vi "ADB-LMS_Esp32.vi"(5 "Monitor Refnum":refnum<vi>, 9 "Serial PID":string, 11 "COM BLE Esp32":refnum<visa-resource-name>) -> (1 "Check  BLE":bool, 2 "CMD Monitor":string="\r\n", 3 "BLE PID Str":string, 4 "Err Open Cnt":u16)   [LabVIEW 2018]
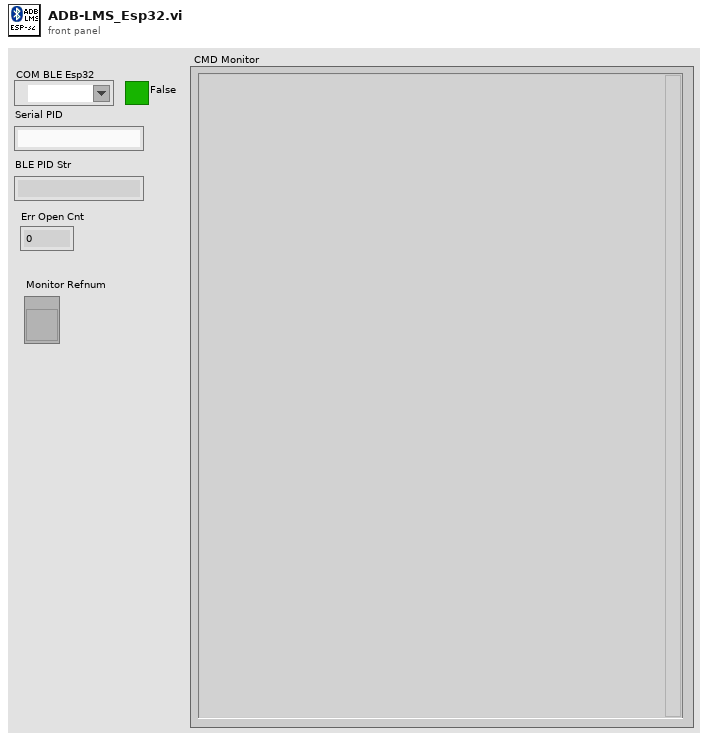
[diagram p1: front panel]
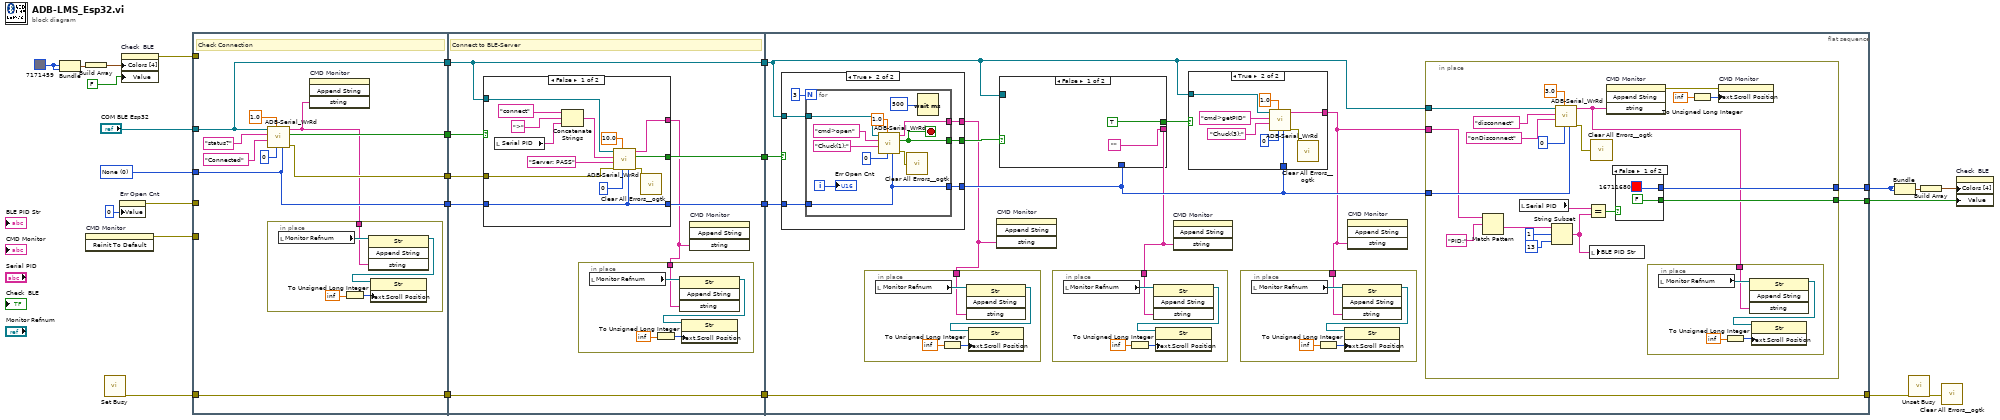
[diagram p0: block diagram]
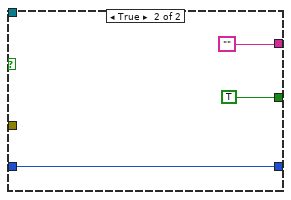
[diagram p2: hidden frame]
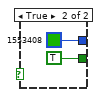
[diagram p3: hidden frame]
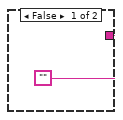
[diagram p4: hidden frame]
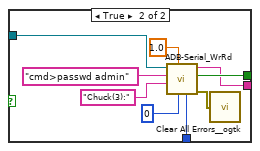
[diagram p5: hidden frame]
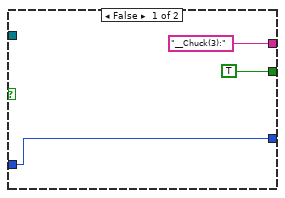
[diagram p6: hidden frame]
diagram:
  w22 = u32 7171459
  w25 = u16 0 items=["None", "XON/XOFF", "RTS/CTS", "XON/XOFF & RTS/CTS", "DTR/DSR", "XON/XOFF & DTR/DSR"] ("flow control (0:none)")
  n1 = Bundle(w22, w22) -> (w23:cluster{u32, u32})  [unwired: 1 in]
  n2 = Build Array(w23) -> (w11:cluster{u32, u32}[])
  n3 = invoke on="CMD Monitor" class="Str" method="Reinit To Default"() -> (error out=w24:errorcluster)  [unwired: 3 in, 2 out]
  n4 = call <vilib>:"Set Busy.vi"() -> ("error out"=w21:errorcluster)  [unwired: 10 in, 1 out]
  n5 = property on="Err Open Cnt" class="DigNum (strict)"("Value"=u16 0 ("Err Open Cnt")) -> (error out=w4:errorcluster)  [unwired: 2 in, 1 out]
  n6 = property on="Check  BLE" class="Bool (strict)"("Colors [4]"=w11, "Value"=FALSE ("Check  BLE")) -> (error out=w12:errorcluster)  [unwired: 2 in, 1 out]
  n7 = flat-sequence {
    tunnel: "COM BLE Esp32" -> [w31]
    tunnel: w25 -> [w29]
    tunnel: w24 -> [_]
    tunnel: w21 -> [w28]
    tunnel: [w32] -> w20
    tunnel: [w31] -> w19
    tunnel: [w30] -> w18
    tunnel: [w29] -> w17
    tunnel: [w28] -> w16
    tunnel: w12 -> [_]
    tunnel: w4 -> [_]
    tunnel: w20 -> [w49]
    tunnel: w19 -> [w44]
    tunnel: w18 -> [w48]
    tunnel: w17 -> [w47]
    tunnel: w16 -> [w45]
    tunnel: [w46] -> w15
    tunnel: [w45] -> w14
    tunnel: [w43] -> w13
    tunnel: [w44] -> w9
    tunnel: [w82] -> w3
    tunnel: w15 -> [w81]
    tunnel: w14 -> [w82]
    tunnel: w13 -> [w80]
    tunnel: w9 -> [w77]
    tunnel: [w76] -> w2
    tunnel: [w75] -> w1
    frame #0 {
      # "Check Connection"
      n8 = call "ADB-Serial_WrRd.vi"("flow control (0:none)"=w29, "Tx Deay"=u16 0, "Timeout(Sec)"=1.0, "PassString"="Connected", "Command"="status?", "ComPort"=w31) -> ("error out"=w30:errorcluster, "PASS"=w32:bool, "received"=w27:string)  [unwired: 3 in]
      n9 = in-place {
        in-place-border: w27 -> [w40]
        n10 = local read "Monitor Refnum"() -> (w41:refnum<vi>)
        n11 = To Unsigned Long Integer(number=inf) -> (unsigned 32bit integer=w37:u32)
        n12 = invoke class="Str" method="Append String"(reference=w41, "string"=w40) -> (reference out=w39:refnum<vi>)  [unwired: 2 in, 3 out]
        n13 = property class="Str"(reference=w39, "Text.Scroll Position"=w37) -> ()  [unwired: 1 in, 2 out]
      }
      n14 = invoke on="CMD Monitor" class="Str" method="Append String"("string"=w27) -> ()  [unwired: 3 in, 4 out]
    }
    frame #1 {
      # "Connect to BLE-Server"
      n15 = case shown="False" w49 {
        tunnel: w44 -> [w66 _]
        tunnel: w48 -> [w64 _]
        tunnel: w47 -> [w59 w68]
        tunnel: [w61 ""] -> w42
        tunnel: [w60 TRUE ("PASS")] -> w46
        tunnel: [w59 w68] -> w43
        frame False {
          n16 = local read "Serial PID"() -> (w55:string)
          n17 = Concatenate Strings("connect" ("Command"), ">", w55) -> (w56:string)
          n18 = call "ADB-Serial_WrRd.vi"("flow control (0:none)"=w59, "Tx Deay"=u16 0, "Timeout(Sec)"=10.0, "error in (no error)"=w64, "PassString"="Server: PASS", "Command"=w56, "ComPort"=w66) -> ("error out"=w63:errorcluster, "PASS"=w60:bool, "received"=w61:string)  [unwired: 2 in]
          n19 = call <userlib>:"Clear All Errors__ogtk.vi"("Error In"=w63) -> ()  [unwired: 3 in, 1 out]
        }
        frame True {
        }
      }
      n20 = in-place {
        in-place-border: w42 -> [w53]
        n21 = local read "Monitor Refnum"() -> (w54:refnum<vi>)
        n22 = To Unsigned Long Integer(number=inf) -> (unsigned 32bit integer=w50:u32)
        n23 = invoke class="Str" method="Append String"(reference=w54, "string"=w53) -> (reference out=w52:refnum<vi>)  [unwired: 2 in, 3 out]
        n24 = property class="Str"(reference=w52, "Text.Scroll Position"=w50) -> ()  [unwired: 1 in, 2 out]
      }
      n25 = invoke on="CMD Monitor" class="Str" method="Append String"("string"=w42) -> ()  [unwired: 3 in, 4 out]
    }
    frame #2 {
      n26 = case shown="True" w81 {
        tunnel: w80 -> [w148 w155]
        tunnel: [TRUE ("PASS") w154] -> w79
        tunnel: ["__Chuck(3):" w153] -> w73
        tunnel: w77 -> [_ w152]
        tunnel: [w148 w151] -> w74
        frame False {
        }
        frame True {
          n27 = for {
            N: 3 -> [_]
            tunnel: w155 -> [w157]
            tunnel: [w162] -> w154
            tunnel: [w160] -> w153
            tunnel: w152 -> [w159]
            tunnel: [w157] -> w151
            i -> [w158]
            stop <- w162 stop-if-true
            n28 = call "ADB-Serial_WrRd.vi"("flow control (0:none)"=w157, "Tx Deay"=u16 0, "Timeout(Sec)"=1.0, "PassString"="Chuck(1):", "Command"="cmd>open", "ComPort"=w159) -> ("error out"=w165:errorcluster, "PASS"=w162:bool, "received"=w160:string)  [unwired: 3 in]
            n29 = call <userlib>:"Clear All Errors__ogtk.vi"("Error In"=w165) -> ()  [unwired: 3 in, 1 out]
            n30 = Wait (ms)(milliseconds to wait=u32 500) -> ()  [unwired: 1 out]
            "Err Open Cnt" <- w158
          }
        }
      }
      n31 = in-place {
        in-place-border: w73 -> [w96]
        n32 = local read "Monitor Refnum"() -> (w97:refnum<vi>)
        n33 = To Unsigned Long Integer(number=inf) -> (unsigned 32bit integer=w93:u32)
        n34 = invoke class="Str" method="Append String"(reference=w97, "string"=w96) -> (reference out=w95:refnum<vi>)  [unwired: 2 in, 3 out]
        n35 = property class="Str"(reference=w95, "Text.Scroll Position"=w93) -> ()  [unwired: 1 in, 2 out]
      }
      n36 = invoke on="CMD Monitor" class="Str" method="Append String"("string"=w73) -> ()  [unwired: 3 in, 4 out]
      n37 = case shown="False" w79 {
        tunnel: w77 -> [_ w144]
        tunnel: w74 -> [_ w141]
        tunnel: [TRUE ("PASS") w140] -> w78
        tunnel: ["" w139] -> w72
        frame False {
        }
        frame True {
          n38 = call "ADB-Serial_WrRd.vi"("flow control (0:none)"=w141, "Tx Deay"=u16 0, "Timeout(Sec)"=1.0, "PassString"="Chuck(3):", "Command"="cmd>passwd admin" ("Write Buffer"), "ComPort"=w144) -> ("error out"=w143:errorcluster, "PASS"=w140:bool, "received"=w139:string)  [unwired: 3 in]
          n39 = call <userlib>:"Clear All Errors__ogtk.vi"("Error In"=w143) -> ()  [unwired: 3 in, 1 out]
        }
      }
      n40 = in-place {
        in-place-border: w72 -> [w91]
        n41 = local read "Monitor Refnum"() -> (w92:refnum<vi>)
        n42 = To Unsigned Long Integer(number=inf) -> (unsigned 32bit integer=w88:u32)
        n43 = invoke class="Str" method="Append String"(reference=w92, "string"=w91) -> (reference out=w90:refnum<vi>)  [unwired: 2 in, 3 out]
        n44 = property class="Str"(reference=w90, "Text.Scroll Position"=w88) -> ()  [unwired: 1 in, 2 out]
      }
      n45 = invoke on="CMD Monitor" class="Str" method="Append String"("string"=w72) -> ()  [unwired: 3 in, 4 out]
      n46 = case shown="True" w78 {
        tunnel: w77 -> [_ w136]
        tunnel: w74 -> [_ w130]
        tunnel: ["" w129] -> w71
        frame False {
        }
        frame True {
          n47 = call "ADB-Serial_WrRd.vi"("flow control (0:none)"=w130, "Tx Deay"=u16 0, "Timeout(Sec)"=1.0, "PassString"="Chuck(3):", "Command"="cmd>getPID" ("Write Buffer"), "ComPort"=w136) -> ("error out"=w132:errorcluster, "received"=w129:string)  [unwired: 3 in, 1 out]
          n48 = call <userlib>:"Clear All Errors__ogtk.vi"("Error In"=w132) -> ()  [unwired: 3 in, 1 out]
        }
      }
      n49 = in-place {
        in-place-border: w71 -> [w86]
        n50 = local read "Monitor Refnum"() -> (w87:refnum<vi>)
        n51 = To Unsigned Long Integer(number=inf) -> (unsigned 32bit integer=w83:u32)
        n52 = invoke class="Str" method="Append String"(reference=w87, "string"=w86) -> (reference out=w85:refnum<vi>)  [unwired: 2 in, 3 out]
        n53 = property class="Str"(reference=w85, "Text.Scroll Position"=w83) -> ()  [unwired: 1 in, 2 out]
      }
      n54 = invoke on="CMD Monitor" class="Str" method="Append String"("string"=w71) -> ()  [unwired: 3 in, 4 out]
      n55 = in-place {
        in-place-border: w77 -> [w117]
        in-place-border: w74 -> [w110]
        in-place-border: w71 -> [w105]
        in-place-border: [w101] -> w76
        in-place-border: [w100] -> w75
        n56 = Match Pattern(string=w105, regular expression="PID:") -> (after substring=w107:string)  [unwired: 1 in, 3 out]
        n57 = local read "Serial PID"() -> (w104:string)
        n58 = String Subset(string=w107, offset (0)=1, length (rest)=13 ("length (rest)")) -> (substring=w103:string)
        n59 = call "ADB-Serial_WrRd.vi"("flow control (0:none)"=w110, "Tx Deay"=u16 0, "Timeout(Sec)"=3.0, "PassString"="onDisconnect", "Command"="disconnect", "ComPort"=w117) -> ("error out"=w113:errorcluster, "received"=w98:string)  [unwired: 3 in, 1 out]
        n60 = Equal?(x=w104, y=w103) -> (x = y?=w102:bool)
        n61 = local write "BLE PID Str"(w103) -> ()
        n62 = call <userlib>:"Clear All Errors__ogtk.vi"("Error In"=w113) -> ()  [unwired: 3 in, 1 out]
        n63 = invoke on="CMD Monitor" class="Str" method="Append String"("string"=w98) -> (error out=w99:errorcluster)  [unwired: 3 in, 3 out]
        n64 = case shown="False" w102 {
          tunnel: [u32 16711680 u32 1553408] -> w101
          tunnel: [FALSE ("Check  BLE") TRUE ("Check  BLE")] -> w100
          frame False {
          }
          frame True {
          }
        }
        n65 = in-place {
          in-place-border: w98 -> [w122]
          n66 = local read "Monitor Refnum"() -> (w123:refnum<vi>)
          n67 = To Unsigned Long Integer(number=inf) -> (unsigned 32bit integer=w119:u32)
          n68 = invoke class="Str" method="Append String"(reference=w123, "string"=w122) -> (reference out=w121:refnum<vi>)  [unwired: 2 in, 3 out]
          n69 = property class="Str"(reference=w121, "Text.Scroll Position"=w119) -> ()  [unwired: 1 in, 2 out]
        }
        n70 = To Unsigned Long Integer(number=inf) -> (unsigned 32bit integer=w111:u32)
        n71 = property on="CMD Monitor" class="Str"(error in=w99, "Text.Scroll Position"=w111) -> ()  [unwired: 1 in, 2 out]
      }
    }
  }
  n72 = Bundle(w2, w2) -> (w7:cluster{u32, u32})  [unwired: 1 in]
  n73 = call <vilib>:"Unset Busy.vi"("error in (no error)"=w3) -> ("error out"=w6:errorcluster)  [unwired: 10 in]
  n74 = Build Array(w7) -> (w8:cluster{u32, u32}[])
  n75 = call <userlib>:"Clear All Errors__ogtk.vi"("Error In"=w6) -> ()  [unwired: 3 in, 1 out]
  n76 = property on="Check  BLE" class="Bool (strict)"("Colors [4]"=w8, "Value"=w1) -> ()  [unwired: 2 in, 2 out]
